vi "Establish_Var2.vi"(11 "SMU Config In":T1) -> (2 "Vname":string, 3 "SMU Config Out":T1, 5 "Execute?":bool)   [LabVIEW 2012]
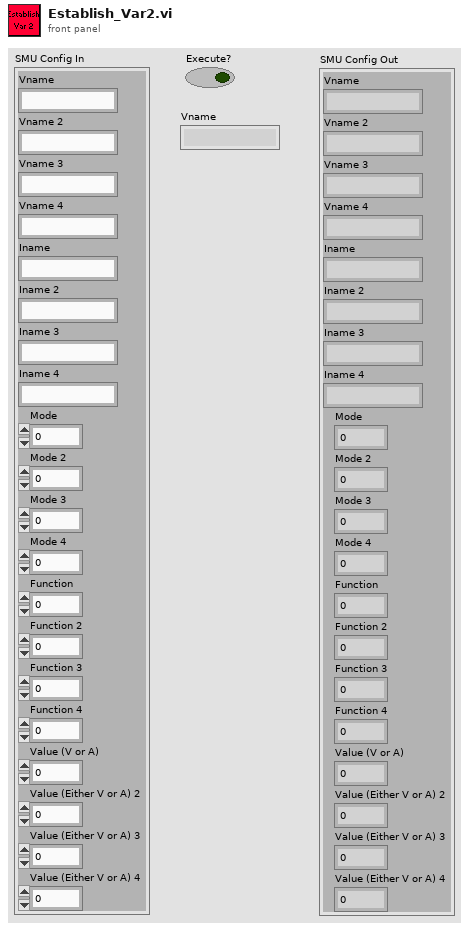
[diagram p1: front panel]
types:
  T1 = cluster{"Vname":string, "Vname 2":string, "Vname 3":string, "Vname 4":string, "Iname":string, "Iname 2":string, "Iname 3":string, "Iname 4":string, "Mode":u16, "Mode 2":u16, "Mode 3":u16, "Mode 4":u16, "Function":u16, "Function 2":u16, "Function 3":u16, "Function 4":u16, "Value (V or A)":dbl, "Value (Either V or A) 2":dbl, "Value (Either V or A) 3":dbl, "Value (Either V or A) 4":dbl}
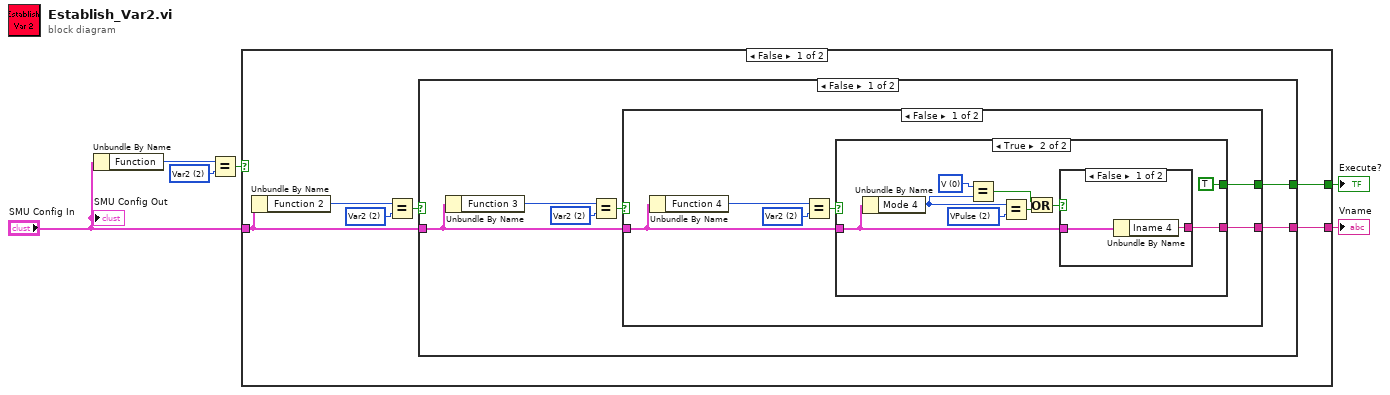
[diagram p0: block diagram]
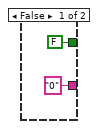
[diagram p2: hidden frame]
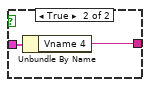
[diagram p3: hidden frame]
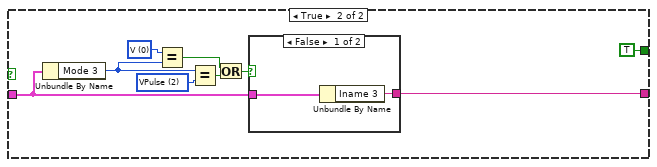
[diagram p4: hidden frame]
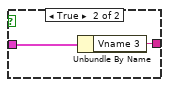
[diagram p5: hidden frame]
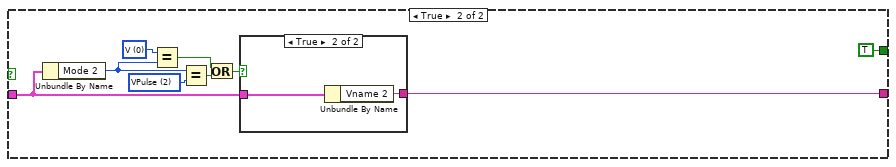
[diagram p6: hidden frame]
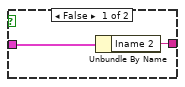
[diagram p7: hidden frame]
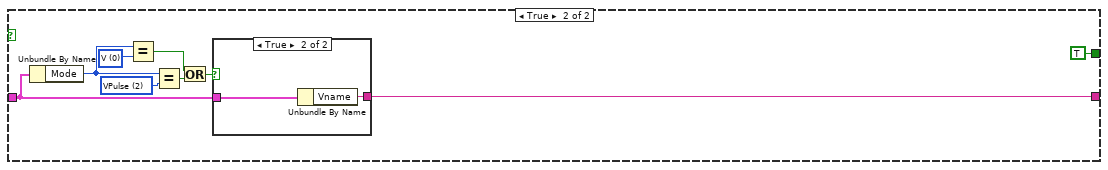
[diagram p8: hidden frame]
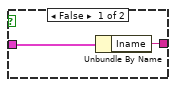
[diagram p9: hidden frame]
diagram:
  w2 = u16 2 items=["disabled", "Var1", "Var2", "Var1'", "Constant"] ("Function")
  n1 = Unbundle By Name("SMU Config In") -> ("Function"=w6:u16)
  n2 = Equal?(x=w6, y=w2) -> (x = y?=w3:bool)
  n3 = case shown="False" w3 {
    tunnel: [w10 w74] -> w4
    tunnel: [w9 TRUE ("x = y?")] -> w5
    tunnel: "SMU Config In" -> [w8 w66]
    frame False {
      w12 = u16 2 items=["disabled", "Var1", "Var2", "Var1'", "Constant"] ("Function")
      n4 = Unbundle By Name(w8) -> ("Function 2"=w7:u16)
      n5 = Equal?(x=w7, y=w12) -> (x = y?=w11:bool)
      n6 = case shown="False" w11 {
        tunnel: [w16 w61] -> w10
        tunnel: [w15 TRUE ("x = y?")] -> w9
        tunnel: w8 -> [w14 w54]
        frame False {
          w18 = u16 2 items=["disabled", "Var1", "Var2", "Var1'", "Constant"] ("Function")
          n7 = Unbundle By Name(w14) -> ("Function 3"=w13:u16)
          n8 = Equal?(x=w13, y=w18) -> (x = y?=w17:bool)
          n9 = case shown="False" w17 {
            tunnel: [w24 w48] -> w16
            tunnel: [w21 TRUE ("x = y?")] -> w15
            tunnel: w14 -> [w20 w40]
            frame False {
              w23 = u16 2 items=["disabled", "Var1", "Var2", "Var1'", "Constant"] ("Function")
              n10 = Unbundle By Name(w20) -> ("Function 4"=w19:u16)
              n11 = Equal?(x=w19, y=w23) -> (x = y?=w22:bool)
              n12 = case shown="True" w22 {
                tunnel: ["0" ("Vname 4") w35] -> w24
                tunnel: [FALSE ("x = y?") TRUE ("x = y?")] -> w21
                tunnel: w20 -> [_ w28]
                frame False {
                }
                frame True {
                  w30 = u16 2 items=["V", "I", "VPulse", "IPulse", "Common"] ("Mode 2")
                  w32 = u16 0 items=["V", "I", "VPulse", "IPulse", "Common"] ("Mode 2")
                  n13 = Unbundle By Name(w28) -> ("Mode 4"=w27:u16)
                  n14 = Equal?(x=w32, y=w27) -> (x = y?=w33:bool)
                  n15 = Equal?(x=w27, y=w30) -> (x = y?=w31:bool)
                  n16 = Or(x=w33, y=w31) -> (x .or. y?=w29:bool)
                  n17 = case shown="False" w29 {
                    tunnel: [w37 w38] -> w35
                    tunnel: w28 -> [w36 w39]
                    frame False {
                      n18 = Unbundle By Name(w36) -> ("Iname 4"=w37:string)
                    }
                    frame True {
                      n19 = Unbundle By Name(w39) -> ("Vname 4"=w38:string)
                    }
                  }
                }
              }
            }
            frame True {
              w44 = u16 2 items=["V", "I", "VPulse", "IPulse", "Common"] ("Mode 2")
              w43 = u16 0 items=["V", "I", "VPulse", "IPulse", "Common"] ("Mode 2")
              n20 = Unbundle By Name(w40) -> ("Mode 3"=w41:u16)
              n21 = Equal?(x=w43, y=w41) -> (x = y?=w46:bool)
              n22 = Equal?(x=w41, y=w44) -> (x = y?=w45:bool)
              n23 = Or(x=w46, y=w45) -> (x .or. y?=w42:bool)
              n24 = case shown="False" w42 {
                tunnel: [w49 w51] -> w48
                tunnel: w40 -> [w50 w52]
                frame False {
                  n25 = Unbundle By Name(w50) -> ("Iname 3"=w49:string)
                }
                frame True {
                  n26 = Unbundle By Name(w52) -> ("Vname 3"=w51:string)
                }
              }
            }
          }
        }
        frame True {
          w56 = u16 2 items=["V", "I", "VPulse", "IPulse", "Common"] ("Mode 2")
          w57 = u16 0 items=["V", "I", "VPulse", "IPulse", "Common"] ("Mode 2")
          n27 = Unbundle By Name(w54) -> ("Mode 2"=w53:u16)
          n28 = Equal?(x=w57, y=w53) -> (x = y?=w59:bool)
          n29 = Equal?(x=w53, y=w56) -> (x = y?=w58:bool)
          n30 = Or(x=w59, y=w58) -> (x .or. y?=w55:bool)
          n31 = case shown="True" w55 {
            tunnel: [w62 w64] -> w61
            tunnel: w54 -> [w63 w65]
            frame False {
              n32 = Unbundle By Name(w63) -> ("Iname 2"=w62:string)
            }
            frame True {
              n33 = Unbundle By Name(w65) -> ("Vname 2"=w64:string)
            }
          }
        }
      }
    }
    frame True {
      w71 = u16 2 items=["V", "I", "VPulse", "IPulse", "Common"] ("Mode")
      w72 = u16 0 items=["V", "I", "VPulse", "IPulse", "Common"] ("Mode")
      n34 = Unbundle By Name(w66) -> ("Mode"=w67:u16)
      n35 = Equal?(x=w67, y=w72) -> (x = y?=w70:bool)
      n36 = Equal?(x=w67, y=w71) -> (x = y?=w69:bool)
      n37 = Or(x=w70, y=w69) -> (x .or. y?=w68:bool)
      n38 = case shown="True" w68 {
        tunnel: [w75 w77] -> w74
        tunnel: w66 -> [w76 w78]
        frame False {
          n39 = Unbundle By Name(w76) -> ("Iname"=w75:string)
        }
        frame True {
          n40 = Unbundle By Name(w78) -> ("Vname"=w77:string)
        }
      }
    }
  }
  "Execute?" <- w5
  "Vname" <- w4
  "SMU Config Out" <- "SMU Config In"
